vi "write to file.vi"() -> ()   [LabVIEW 2011]
panel:
  in  "number of acquisitions":i32=10 min=1 max=100
  out "data":sgl[](graph)
  in  "number of points/acquisition":i32=10
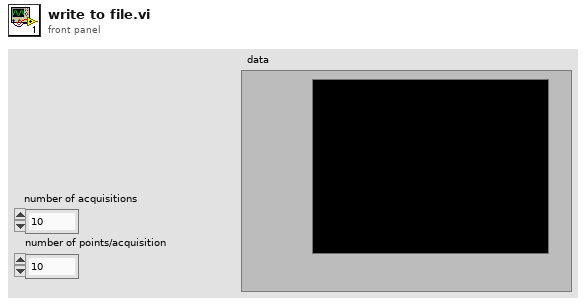
[diagram p1: front panel]
types:
  T1 = enum16{"open", "replace", "create", "open or create", "replace or create", "replace or create with confirmation"}
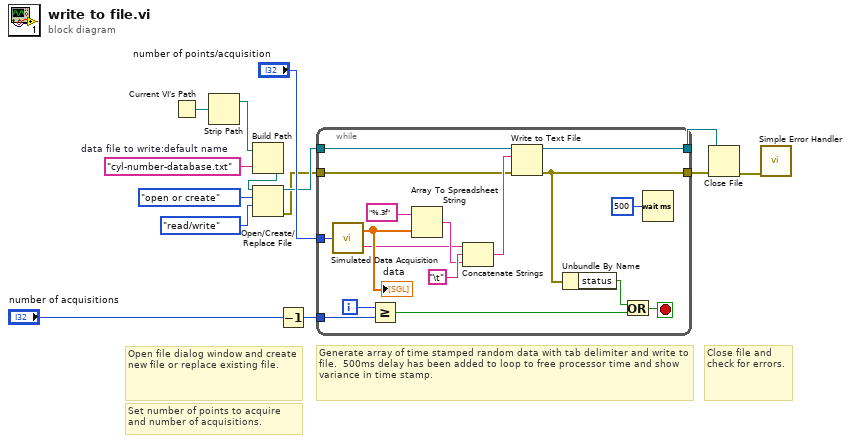
[diagram p0: block diagram]
diagram:
  w3 = "cyl-number-database.txt"  # data file to write:default name
  # "Close file and \ncheck for errors."
  # "Generate array of time stamped random data with tab delimiter and write to file.  500ms delay has been added to loop to free processor time and show variance in time stamp."
  # "Set number of points to acquire and number of acquisitions."
  # "Open file dialog window and create new file or replace existing file."
  n1 = Current VI's Path() -> (path=w2:path)
  n2 = Strip Path(path=w2) -> (stripped path=w1:path)  [unwired: 1 out]
  n3 = Build Path(base path=w1, name or relative path=w3) -> (appended path=w4:path)
  n4 = Open/Create/Replace File(file path (use dialog)=w4, operation (0:open)=T1."open or create", access (0:read/write)=enum16{"read/write", "read-only", "write-only"}."read/write") -> (refnum out=w8:refnum<file>, error out=w7:errorcluster)  [unwired: 1 in, 3 out]
  n5 = Decrement(x="number of acquisitions") -> (x-1=w9:i32)
  n6 = while {
    tunnel: [w21] -> w13
    tunnel: [w20] -> w12
    tunnel: "number of points/acquisition" -> [w31]
    tunnel: w9 -> [w17]
    tunnel: w8 -> [w16]
    tunnel: w7 -> [w15]
    i -> [w26]
    stop <- w25 stop-if-true
    n7 = call "Simulated Data Acquisition.vi"("# of points"=w31) -> ("data"=w23:sgl[], "time"=w22:string)
    "data" <- w23
    n8 = Greater Or Equal?(x=w26, y=w17) -> (x >= y?=w27:bool)
    n9 = Array To Spreadsheet String(array=w23, 3:"%.3f") -> (spreadsheet string=w29:string)  [unwired: 1 out]
    n10 = Concatenate Strings(w22, "\t" ("Tab"), w29) -> (w19:string)
    n11 = Write to Text File(file (use dialog)=w16, text=w19, error in=w15) -> (refnum out=w21:refnum<file>, error out=w20:errorcluster)  [unwired: 1 in, 1 out]
    n12 = Unbundle By Name(w20) -> ("status"=w28:bool)
    n13 = Or(x=w28, y=w27) -> (x .or. y?=w25:bool)
    n14 = Wait (ms)(milliseconds to wait=u32 500 ("millisecond multiple")) -> ()  [unwired: 1 out]
  }
  n15 = Close File(refnum=w13, error in=w12) -> (error out=w11:errorcluster)  [unwired: 1 out]
  n16 = call <vilib>:"Simple Error Handler.vi"("error in (no error)"=w11) -> ()  [unwired: 1 in, 8 out]
